vi "TouchPanel.NumericGui.vi"(4 "Password Display (F)":bool, 6 "Max Length (70)":i32=70, 8 "Integer (F)":bool, 9 "empty visible (F)":bool caption="empty visilbe (F)", 10 "Numeric In":ext, 11 "Message In":string) -> (1 "Canceled":bool, 2 "Numeric Out":ext)   [LabVIEW 2016]
uses:
  TouchPanel.DriverCommands.ctl
  Translator/Translator.Global.vi
panel:
  in  "Empty":bool
  in  "~-Inf":bool caption="-Inf"
  in  "~+Inf":bool caption="+Inf"
  out "Text 2":string
  out "_tab":enum32{"Keyboard", "Arrows"}(tab)
  in  "~.":bool
  in  "~0":bool
  in  "~9":bool
  in  "~8":bool
  in  "~7":bool
  in  "~6":bool
  in  "~5":bool
  in  "~4":bool
  in  "~3":bool
  in  "~2":bool
  in  "~1":bool
  in  "~UP":bool
  in  "~Down":bool
  in  "~-":bool caption="-"
  in  "~+":bool caption="+"
  in  "~Right":bool
  in  "~Left":bool
  in  "Clear":bool
  in  "~+/-":bool
  out "Message":string
  in  "OKButton":bool
  in  "CancelButton":bool
  in  "Text":string
  in  "Delete":bool
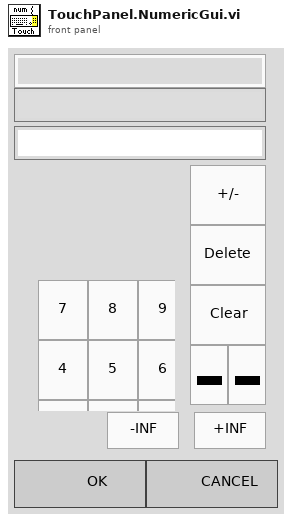
[diagram p1: front panel]
types:
  T1 = typedef "TouchPanel.DriverCommands.ctl" = enum16{"No Command", "Initialize", "Add Character", "Replace Character", "Delete Character", "Move Left", "Move Right", "Update Edit Position"}
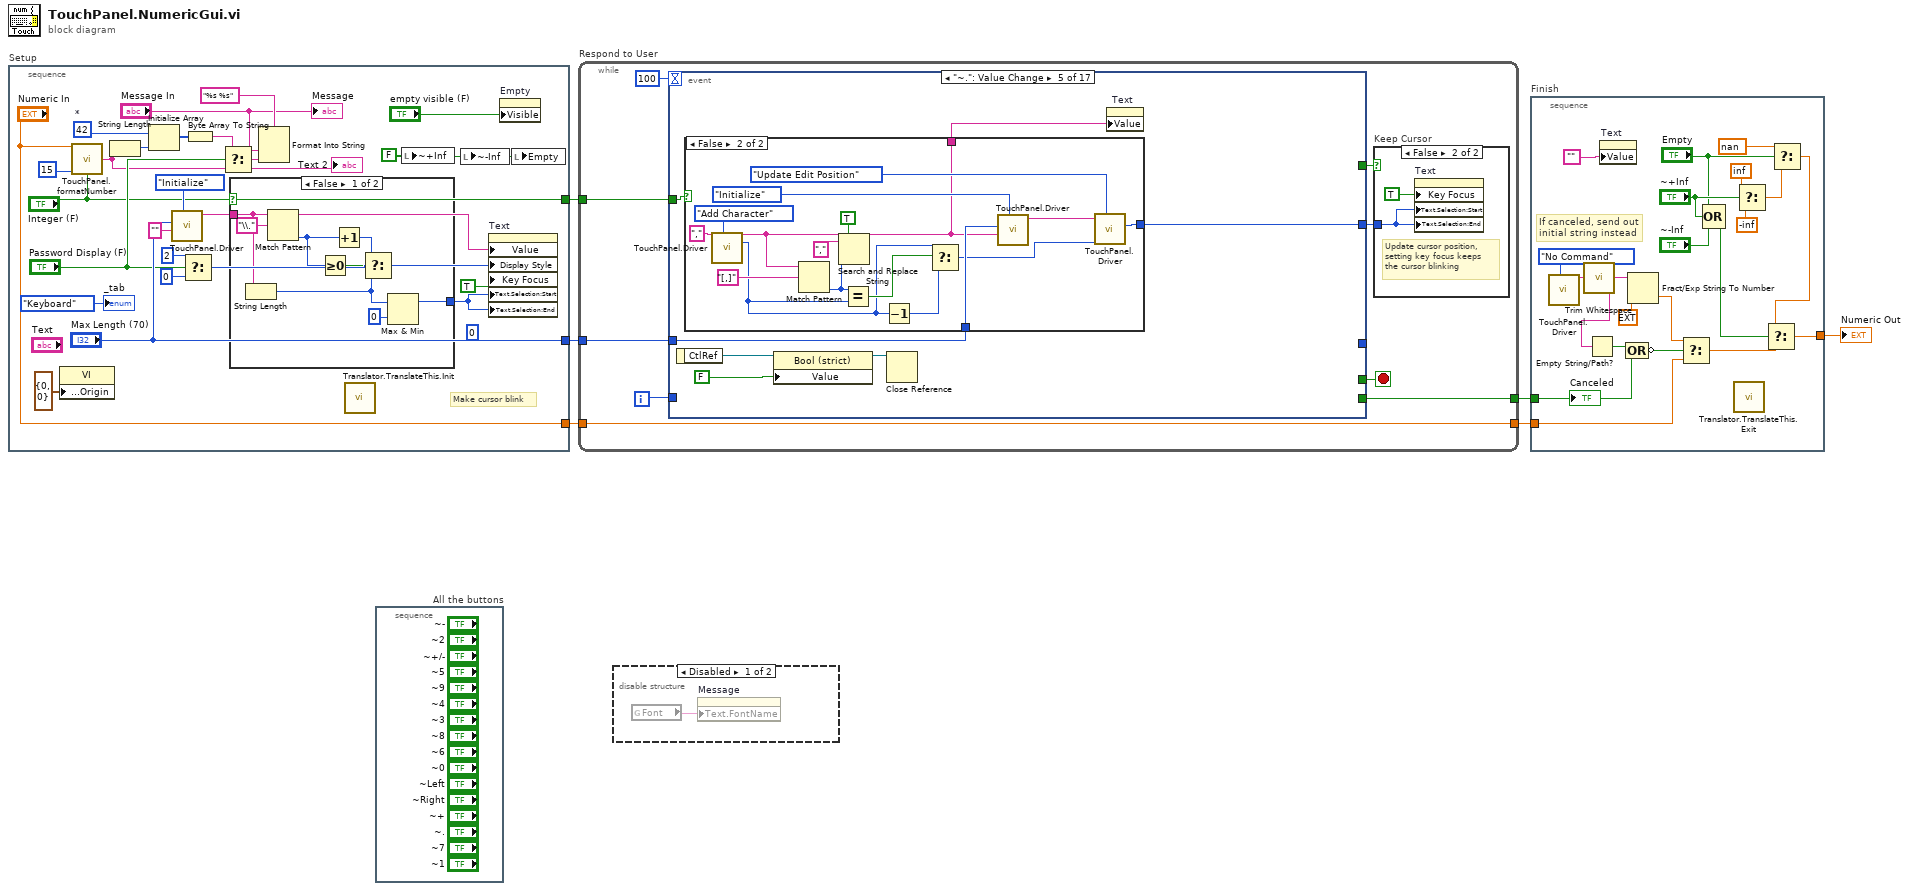
[diagram p0: block diagram]
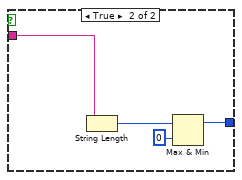
[diagram p3: hidden frame]
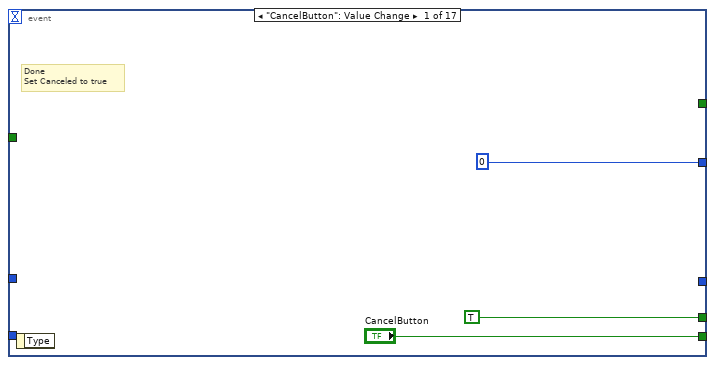
[diagram p5: hidden frame]
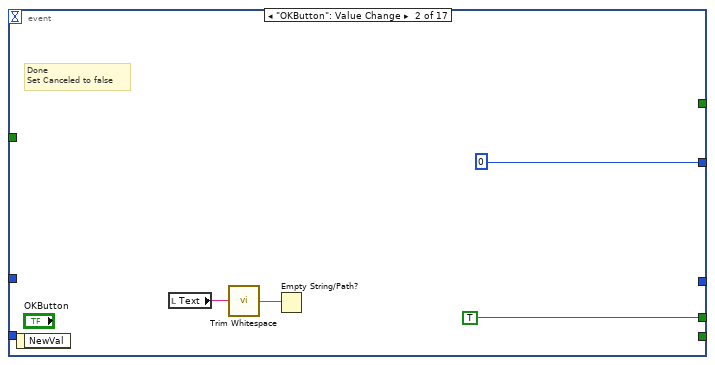
[diagram p6: hidden frame]
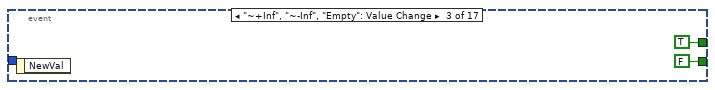
[diagram p7: hidden frame]
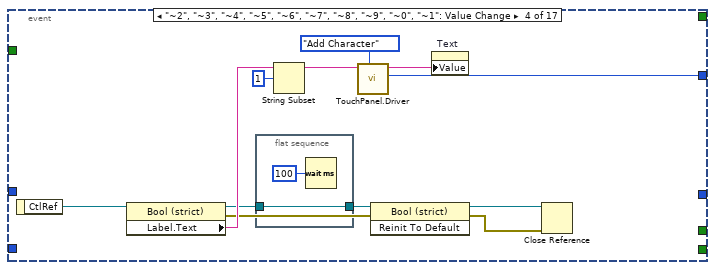
[diagram p8: hidden frame]
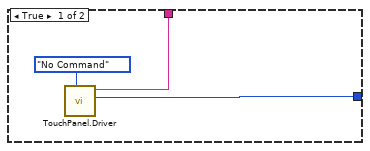
[diagram p9: hidden frame]
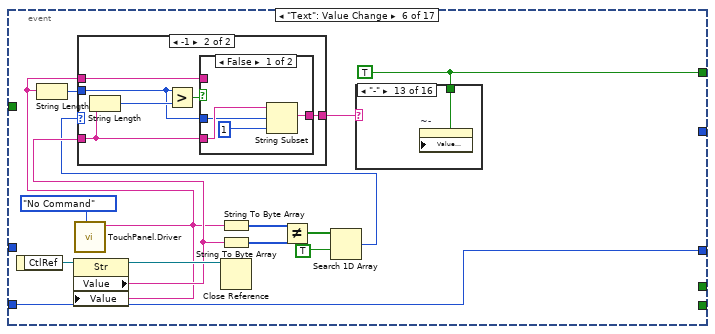
[diagram p10: hidden frame]
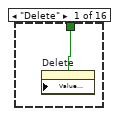
[diagram p11: hidden frame]
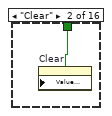
[diagram p12: hidden frame]
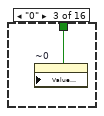
[diagram p13: hidden frame]
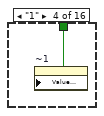
[diagram p14: hidden frame]
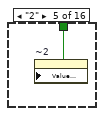
[diagram p15: hidden frame]
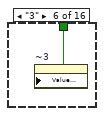
[diagram p16: hidden frame]
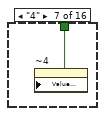
[diagram p17: hidden frame]
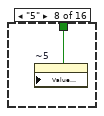
[diagram p18: hidden frame]
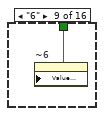
[diagram p19: hidden frame]
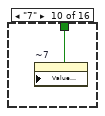
[diagram p20: hidden frame]
diagram:
  n1 = stacked-sequence "Setup" {
    tunnel: ["Numeric In"] -> w6
    tunnel: ["Max Length (70)"] -> w3
    tunnel: ["Integer (F)"] -> w2
    frame #0 {
      w8 = FALSE ("+Inf")
      (unwired) u32 0 ("Text.Selection:End")
      w19 = u8 42  # *
      # "Make cursor blink"
      n2 = property class="VI"("Front Panel Window:Origin"=cluster{"Horizontal":i16, "Vertical":i16} {"Horizontal"=0, "Vertical"=0}) -> ()  [unwired: 2 in, 2 out]
      n3 = call "TouchPanel.formatNumber.vi"("number in"="Numeric In", "significant digits (6)"=i16 15, "Integer (F)"="Integer (F)") -> ("string out"=w9:string)  [unwired: 1 in, 11 out]
      "Text 2" <- w9
      n4 = String Length(string=w9) -> (length=w20:i32)
      n5 = Initialize Array(w19, w20) -> (w18:u8[])
      n6 = call "TouchPanel.Driver.vi"("Driver Commands"=TouchPanel.DriverCommands."Initialize", "Initial String"="", "Max Length (70)"="Max Length (70)") -> ("String Out"=w12:string)  [unwired: 2 in, 6 out]
      n7 = Select(t=u32 2 ("Display Style"), s="Password Display (F)", f=u32 0 ("Display Style")) -> (s? t:f=w28:u32)
      n8 = Byte Array To String(unsigned byte array=w18) -> (string=w17:string)
      n9 = Select(t=w17, s="Password Display (F)", f=w9) -> (s? t:f=w22:string)
      n10 = case shown="False" "Integer (F)" {
        tunnel: w12 -> [w37 w43]
        tunnel: [w35 w42] -> w11
        frame False {
          n11 = String Length(string=w37) -> (length=w32:i32)
          n12 = Match Pattern(string=w37, regular expression="\\.") -> (offset past match=w34:i32)  [unwired: 4 out]
          n13 = Greater Or Equal To 0?(x=w34) -> (x >= 0?=w38:bool)
          n14 = Increment(x=w34) -> (x+1=w33:i32)
          n15 = Select(t=w33, s=w38, f=w32) -> ()  [unwired: 1 out]
          n16 = Max & Min(x=w32, y=0 ("Text.Selection:End")) -> (max(x,y)=w35:i32)  [unwired: 1 out]
        }
        frame True {
          n17 = String Length(string=w43) -> (length=w40:i32)
          n18 = Max & Min(x=w40, y=0 ("Text.Selection:End")) -> (max(x,y)=w42:i32)  [unwired: 1 out]
        }
      }
      n19 = Format Into String(format string="%s %s", "Message In", w22) -> ()  [unwired: 2 in, 2 out]
      n20 = call "Translator.TranslateThis.Init.vi"() -> ()  [unwired: 11 in, 1 out]
      n21 = local write "~+Inf"(w8) -> ()
      n22 = local write "~-Inf"(w8) -> ()
      n23 = property on="Text" class="Str"("Value"=w12, "Display Style"=w28, "Key Focus"=TRUE, "Text.Selection:Start"=w11, "Text.Selection:End"=w11) -> ()  [unwired: 2 in, 2 out]
      n24 = property on="Empty" class="Bool (strict)"("Visible"="empty visible (F)") -> ()  [unwired: 2 in, 2 out]
      n25 = local write "Empty"(w8) -> ()
      "Message" <- "Message In"
      "_tab" <- enum32{"Keyboard", "Arrows"}."Keyboard" ("_tab")
    }
  }
  n26 = stacked-sequence "All the buttons" {
    frame #0 {
    }
  }
  n27 = while "Respond to User" {
    tunnel: w6 -> [w49]
    tunnel: [w50] -> w5
    tunnel: [w49] -> w4
    tunnel: w3 -> [w48]
    tunnel: w2 -> [w44]
    i -> [w45]
    stop <- w52 stop-if-true
    n28 = event shown="[4] \"~.\": Value Change" {
      selector: _ -> [_ _ _ _ _ _ _ _ _ _ _ _ _ _ _ _ _]
      dyn-events: _ -> [_ _ _ _ _ _ _ _ _ _ _ _ _ _ _ _ _]
      timeout: 100 -> [_ _ _ _ _ _ _ _ _ _ _ _ _ _ _ _ _]
      tunnel: [TRUE TRUE TRUE _ _ _ _ _ _ _ _ _ _ _ _ _ _] -> w52
      tunnel: [0 ("Edit Position") 0 ("Edit Position") _ w72 w84 _ _ w173 w198 w220 u32 0 ("Text.Selection Start") w241 w263 w273 w337 w401 w403] -> w51
      tunnel: ["CancelButton" _ FALSE ("Cancel") _ _ _ _ _ _ _ _ _ _ _ _ _ _] -> w50
      tunnel: w48 -> [_ _ _ _ w83 _ _ w176 w201 w223 w238 _ _ w294 w360 _ _]
      tunnel: [_ _ _ _ _ w108 TRUE _ _ _ _ _ _ _ _ _ _] -> w47
      tunnel: w45 -> [_ _ _ _ _ w107 _ _ _ _ _ _ _ _ _ _ _]
      tunnel: [_ _ _ _ _ w107 _ _ _ _ _ _ _ _ _ _ _] -> _
      tunnel: w44 -> [_ _ _ _ w78 _ _ _ _ _ _ _ _ w286 w351 _ _]
      event "CancelButton": Value Change {
        # "Done\nSet Canceled to true"
        n29 = event-data() -> ()  [unwired: 2 out]
      }
      event "OKButton": Value Change {
        # "Done\nSet Canceled to false"
        n30 = event-data() -> ()  [unwired: 2 out]
        n31 = local read "Text"() -> (w58:string)
        n32 = call <vilib>:"Trim Whitespace.vi"("string"=w58) -> ("trimmed string"=w59:string)  [unwired: 1 in]
        n33 = Empty String/Path?(string/path=w59) -> ()  [unwired: 1 out]
      }
      event "~+Inf", "~-Inf", "Empty": Value Change {
        n34 = event-data() -> ()  [unwired: 2 out]
      }
      event "~2", "~3", "~4", "~5", "~6", "~7", "~8", "~9", "~0", "~1": Value Change {
        n35 = event-data() -> ("CtlRef"=w75:refnum<vi>)  [unwired: 1 out]
        n36 = property class="Bool (strict)"(reference=w75) -> (reference out=w67:refnum<vi>, error out=w65:errorcluster, "Label.Text"=w73:string)  [unwired: 1 in]
        n37 = flat-sequence {
          tunnel: [w77] -> w66
          tunnel: w67 -> [w77]
          frame #0 {
            n38 = Wait (ms)(milliseconds to wait=u32 100) -> ()  [unwired: 1 out]
          }
        }
        n39 = String Subset(string=w73, offset (0)=1) -> (substring=w70:string)  [unwired: 1 in]
        n40 = call "TouchPanel.Driver.vi"("Driver Commands"=TouchPanel.DriverCommands."Add Character", "Character"=w70) -> ("Edit Position"=w72:i32, "String Out"=w71:string)  [unwired: 3 in, 5 out]
        n41 = invoke class="Bool (strict)" method="Reinit To Default"(reference=w66, error in=w65) -> (reference out=w68:refnum<vi>, error out=w64:errorcluster)  [unwired: 1 in, 1 out]
        n42 = property on="Text" class="Str"("Value"=w71) -> ()  [unwired: 2 in, 2 out]
        n43 = Close Reference(reference=w68, error in (no error)=w64) -> ()  [unwired: 1 out]
      }
      event "~.": Value Change {
        n44 = event-data() -> ("CtlRef"=w80:refnum<vi>)  [unwired: 1 out]
        n45 = case shown="False" w78 {
          tunnel: [w86 w101] -> w84
          tunnel: w83 -> [_ w100]
          tunnel: [w85 w88] -> w79
          frame True {
            n46 = call "TouchPanel.Driver.vi"("Driver Commands"=TouchPanel.DriverCommands."No Command") -> ("Edit Position"=w86:i32, "String Out"=w85:string)  [unwired: 4 in, 5 out]
          }
          frame False {
            n47 = call "TouchPanel.Driver.vi"("Driver Commands"=TouchPanel.DriverCommands."Add Character", "Character"=",") -> ("Edit Position"=w90:i32, "String Out"=w96:string)  [unwired: 3 in, 5 out]
            n48 = Match Pattern(string=w96, regular expression="[,]") -> (offset past match=w92:i32)  [unwired: 4 out]
            n49 = Search and Replace String(replace all?=TRUE ("replace all? (F)"), input string=w96, search string="," ("Character"), offset=w92) -> (result string=w88:string)  [unwired: 1 in, 6 out]
            n50 = Equal?(x=w92, y=w90) -> (x = y?=w91:bool)
            n51 = Decrement(x=w90) -> (x-1=w89:i32)
            n52 = Select(t=w90, s=w91, f=w89) -> (s? t:f=w93:i32)
            n53 = call "TouchPanel.Driver.vi"("Driver Commands"=TouchPanel.DriverCommands."Initialize", "Initial String"=w88, "Max Length (70)"=w100) -> ("String Out"=w103:string)  [unwired: 2 in, 6 out]
            n54 = call "TouchPanel.Driver.vi"("Driver Commands"=TouchPanel.DriverCommands."Update Edit Position", "New Edit Position"=w93, "Character"=w103) -> ("Edit Position"=w101:i32)  [unwired: 2 in, 6 out]
          }
        }
        n55 = property class="Bool (strict)"(reference=w80, "Value"=FALSE) -> (reference out=w82:refnum<vi>)  [unwired: 1 in, 1 out]
        n56 = Close Reference(reference=w82) -> ()  [unwired: 1 in, 1 out]
        n57 = property on="Text" class="Str"("Value"=w79) -> ()  [unwired: 2 in, 2 out]
      }
      event "Text": Value Change {
        w108 = TRUE
        n58 = event-data() -> ("CtlRef"=w118:refnum<vi>)  [unwired: 1 out]
        n59 = call "TouchPanel.Driver.vi"("Driver Commands"=TouchPanel.DriverCommands."No Command") -> ("String Out"=w106:string)  [unwired: 4 in, 6 out]
        n60 = String Length(string=w106) -> (length=w115:i32)
        n61 = property class="Str"(reference=w118, "Value"=w106) -> (reference out=w117:refnum<vi>, "Value"=w111:string)  [unwired: 1 in, 1 out]
        n62 = String To Byte Array(string=w106) -> (unsigned byte array=w112:u8[])
        n63 = String To Byte Array(string=w111) -> (unsigned byte array=w113:u8[])
        n64 = Close Reference(reference=w117) -> ()  [unwired: 1 in, 1 out]
        n65 = Not Equal?(x=w112, y=w113) -> (x != y?=w110:bool[])
        n66 = Search 1D Array(1D array=w110, element=TRUE) -> (index of element=w105:i32)  [unwired: 1 out]
        n67 = case shown="-1" w105 {
          selector: w105 -> [w135 _]
          tunnel: w106 -> [w137 w150]
          tunnel: w111 -> [w136 w149]
          tunnel: w115 -> [w139 w146]
          tunnel: [w134 w148] -> w109
          frame Default {
            n68 = String Length(string=w136) -> (length=w140:i32)
            n69 = Greater?(x=w139, y=w140) -> (0:w138:bool)
            n70 = case shown="False" w138 {
              tunnel: w137 -> [_ _]
              tunnel: w136 -> [w144 _]
              tunnel: w135 -> [w143 _]
              tunnel: [w141 "Delete" ("Value")] -> w134
              frame False {
                n71 = String Subset(string=w144, offset (0)=w143, length (rest)=1 ("length (rest)")) -> (substring=w141:string)
              }
              frame True {
              }
            }
          }
          frame -1 {
            n72 = String Length(string=w149) -> (length=w147:i32)
            n73 = Greater?(x=w146, y=w147) -> (0:w151:bool)
            n74 = case shown="False" w151 {
              tunnel: w150 -> [_ _]
              tunnel: w149 -> [w155 _]
              tunnel: w146 -> [w154 _]
              tunnel: [w152 "Delete" ("Value")] -> w148
              frame False {
                n75 = String Subset(string=w155, offset (0)=w154, length (rest)=1 ("length (rest)")) -> (substring=w152:string)
              }
              frame True {
              }
            }
          }
        }
        n76 = case shown="\"-\"" w109 {
          tunnel: w108 -> [w119 w120 w121 w122 w123 w124 w125 w126 w127 w128 w129 w130 w131 w132 w133 _]
          frame "Delete" {
            n77 = property on="Delete" class="Bool (strict)"("Value (Signaling)"=w119) -> ()  [unwired: 2 in, 2 out]
          }
          frame "Clear" {
            n78 = property on="Clear" class="Bool (strict)"("Value (Signaling)"=w120) -> ()  [unwired: 2 in, 2 out]
          }
          frame "0" {
            n79 = property on="~0" class="Bool (strict)"("Value (Signaling)"=w121) -> ()  [unwired: 2 in, 2 out]
          }
          frame "1" {
            n80 = property on="~1" class="Bool (strict)"("Value (Signaling)"=w122) -> ()  [unwired: 2 in, 2 out]
          }
          frame "2" {
            n81 = property on="~2" class="Bool (strict)"("Value (Signaling)"=w123) -> ()  [unwired: 2 in, 2 out]
          }
          frame "3" {
            n82 = property on="~3" class="Bool (strict)"("Value (Signaling)"=w124) -> ()  [unwired: 2 in, 2 out]
          }
          frame "4" {
            n83 = property on="~4" class="Bool (strict)"("Value (Signaling)"=w125) -> ()  [unwired: 2 in, 2 out]
          }
          frame "5" {
            n84 = property on="~5" class="Bool (strict)"("Value (Signaling)"=w126) -> ()  [unwired: 2 in, 2 out]
          }
          frame "6" {
            n85 = property on="~6" class="Bool (strict)"("Value (Signaling)"=w127) -> ()  [unwired: 2 in, 2 out]
          }
          frame "7" {
            n86 = property on="~7" class="Bool (strict)"("Value (Signaling)"=w128) -> ()  [unwired: 2 in, 2 out]
          }
          frame "8" {
            n87 = property on="~8" class="Bool (strict)"("Value (Signaling)"=w129) -> ()  [unwired: 2 in, 2 out]
          }
          frame "9" {
            n88 = property on="~9" class="Bool (strict)"("Value (Signaling)"=w130) -> ()  [unwired: 2 in, 2 out]
          }
          frame "-" {
            n89 = property on="~-" class="Bool (strict)"("Value (Signaling)"=w131) -> ()  [unwired: 2 in, 2 out]
          }
          frame "+" {
            n90 = property on="~+" class="Bool (strict)"("Value (Signaling)"=w132) -> ()  [unwired: 2 in, 2 out]
          }
          frame "." {
            n91 = property on="~." class="Bool (strict)"("Value (Signaling)"=w133) -> ()  [unwired: 2 in, 2 out]
          }
          frame Default {
          }
        }
      }
      event Timeout {
        n92 = event-data() -> ()  [unwired: 2 out]
        n93 = property on="Text" class="Str"() -> ("Text.Selection:Start"=w158:u32)  [unwired: 2 in, 2 out]
        n94 = call "TouchPanel.Driver.vi"("Driver Commands"=TouchPanel.DriverCommands."No Command") -> ("Edit Position"=w160:i32)  [unwired: 4 in, 6 out]
        n95 = Not Equal?(x=w160, y=w158) -> (x != y?=w159:bool)
        n96 = case shown="True" w159 {
          tunnel: w158 -> [_ w162]
          frame False {
          }
          frame True {
            n97 = call "TouchPanel.Driver.vi"("Driver Commands"=TouchPanel.DriverCommands."Update Edit Position", "New Edit Position"=w162) -> ()  [unwired: 3 in, 7 out]
          }
        }
      }
      event "~+/-": Value Change {
        w170 = "-" ("regular expression")
        n98 = event-data() -> ("CtlRef"=w166:refnum<vi>)  [unwired: 1 out]
        n99 = property on="Text" class="Str"() -> ("Value"=w171:string, "Text.Selection:Start"=w169:u32)  [unwired: 2 in, 2 out]
        n100 = property class="Bool (strict)"(reference=w166, "Value"=FALSE) -> (reference out=w168:refnum<vi>)  [unwired: 1 in, 1 out]
        n101 = Match Pattern(string=w171, regular expression=w170) -> (offset past match=w172:i32)  [unwired: 4 out]
        n102 = Close Reference(reference=w168) -> ()  [unwired: 1 in, 1 out]
        n103 = case shown="Default" w172 {
          selector: w172 -> [w180 _]
          tunnel: w171 -> [w182 w187]
          tunnel: w170 -> [_ w186]
          tunnel: w169 -> [w181 w185]
          tunnel: [w179 w184] -> w164
          tunnel: [w178 w183] -> w165
          frame Default {
            n104 = String Subset(string=w182, offset (0)=w180) -> (substring=w178:string)  [unwired: 1 out]
            n105 = Subtract(x=w181, y=w180) -> (x-y=w179:u32)
          }
          frame -1 {
            n106 = Increment(x=w185) -> (x+1=w184:u32)
            n107 = Concatenate Strings(w186, w187) -> (w183:string)
          }
        }
        n108 = call "TouchPanel.Driver.vi"("Driver Commands"=TouchPanel.DriverCommands."Initialize", "Initial String"=w165, "Max Length (70)"=w176) -> ("String Out"=w175:string)  [unwired: 2 in, 6 out]
        n109 = property on="Text" class="Str"("Value"=w165) -> ()  [unwired: 2 in, 2 out]
        n110 = call "TouchPanel.Driver.vi"("Driver Commands"=TouchPanel.DriverCommands."Update Edit Position", "New Edit Position"=w164, "Character"=w175) -> ("Edit Position"=w173:i32)  [unwired: 2 in, 6 out]
      }
      event "~+": Value Change {
        w196 = "-" ("regular expression")
        n111 = event-data() -> ("CtlRef"=w193:refnum<vi>)  [unwired: 1 out]
        n112 = call "TouchPanel.Driver.vi"("Driver Commands"=TouchPanel.DriverCommands."No Command") -> ("Edit Position"=w190:i32, "String Out"=w191:string)  [unwired: 4 in, 5 out]
        n113 = property class="Bool (strict)"(reference=w193, "Value"=FALSE) -> (reference out=w195:refnum<vi>)  [unwired: 1 in, 1 out]
        n114 = Match Pattern(string=w191, regular expression=w196) -> (offset past match=w197:i32)  [unwired: 4 out]
        n115 = Close Reference(reference=w195) -> ()  [unwired: 1 in, 1 out]
        n116 = case shown="Default" w197 {
          selector: w197 -> [w205 _]
          tunnel: w191 -> [w207 w209]
          tunnel: w196 -> [_ _]
          tunnel: w190 -> [w206 w208]
          tunnel: [w204 w208] -> w188
          tunnel: [w203 w209] -> w189
          frame Default {
            n117 = Subtract(x=w206, y=w205) -> (x-y=w204:i32)
            n118 = String Subset(string=w207, offset (0)=w205) -> (substring=w203:string)  [unwired: 1 out]
          }
          frame -1 {
          }
        }
        n119 = call "TouchPanel.Driver.vi"("Driver Commands"=TouchPanel.DriverCommands."Initialize", "Initial String"=w189, "Max Length (70)"=w201) -> ("String Out"=w200:string)  [unwired: 2 in, 6 out]
        n120 = property on="Text" class="Str"("Value"=w189) -> ()  [unwired: 2 in, 2 out]
        n121 = call "TouchPanel.Driver.vi"("Driver Commands"=TouchPanel.DriverCommands."Update Edit Position", "New Edit Position"=w188, "Character"=w200) -> ("Edit Position"=w198:i32)  [unwired: 2 in, 6 out]
      }
      event "~-": Value Change {
        w218 = "-" ("regular expression")
        n122 = event-data() -> ("CtlRef"=w215:refnum<vi>)  [unwired: 1 out]
        n123 = call "TouchPanel.Driver.vi"("Driver Commands"=TouchPanel.DriverCommands."No Command") -> ("Edit Position"=w212:i32, "String Out"=w213:string)  [unwired: 4 in, 5 out]
        n124 = property class="Bool (strict)"(reference=w215, "Value"=FALSE) -> (reference out=w217:refnum<vi>)  [unwired: 1 in, 1 out]
        n125 = Match Pattern(string=w213, regular expression=w218) -> (offset past match=w219:i32)  [unwired: 4 out]
        n126 = Close Reference(reference=w217) -> ()  [unwired: 1 in, 1 out]
        n127 = case shown="-1" w219 {
          tunnel: w213 -> [w226 w231]
          tunnel: w218 -> [_ w230]
          tunnel: w212 -> [w225 w229]
          tunnel: [w226 w228] -> w211
          tunnel: [w225 w227] -> w210
          frame Default {
          }
          frame -1 {
            n128 = Increment(x=w229) -> (x+1=w227:i32)
            n129 = Concatenate Strings(w230, w231) -> (w228:string)
          }
        }
        n130 = call "TouchPanel.Driver.vi"("Driver Commands"=TouchPanel.DriverCommands."Initialize", "Initial String"=w211, "Max Length (70)"=w223) -> ("String Out"=w222:string)  [unwired: 2 in, 6 out]
        n131 = property on="Text" class="Str"("Value"=w211) -> ()  [unwired: 2 in, 2 out]
        n132 = call "TouchPanel.Driver.vi"("Driver Commands"=TouchPanel.DriverCommands."Update Edit Position", "New Edit Position"=w210, "Character"=w222) -> ("Edit Position"=w220:i32)  [unwired: 2 in, 6 out]
      }
      event "Clear": Value Change {
        n133 = event-data() -> ("CtlRef"=w234:refnum<vi>)  [unwired: 1 out]
        n134 = property class="Bool (strict)"(reference=w234, "Value"=FALSE) -> (reference out=w236:refnum<vi>)  [unwired: 1 in, 1 out]
        n135 = call "TouchPanel.Driver.vi"("Driver Commands"=TouchPanel.DriverCommands."Initialize", "Initial String"="", "Max Length (70)"=w238) -> ("String Out"=w237:string)  [unwired: 2 in, 6 out]
        n136 = Close Reference(reference=w236) -> ()  [unwired: 1 in, 1 out]
        n137 = property on="Text" class="Str"("Value"=w237) -> ()  [unwired: 2 in, 2 out]
      }
      event "~Left": Value Change {
        w243 = 1 ("length (rest)")
        n138 = event-data() -> ("CtlRef"=w250:refnum<vi>)  [unwired: 1 out]
        n139 = property on="Text" class="Str"() -> ("Value"=w249:string, "Text.Selection Start"=w240:u32)  [unwired: 2 in, 2 out]
        n140 = property class="Bool (strict)"(reference=w250, "Value"=FALSE) -> (reference out=w252:refnum<vi>)  [unwired: 1 in, 1 out]
        n141 = String Subset(string=w249, offset (0)=0, length (rest)=w243) -> (substring=w247:string)
        n142 = Equal?(x=w243, y=w240) -> (x = y?=w245:bool)
        n143 = Equal?(x="-", y=w247) -> (x = y?=w244:bool)
        n144 = Compound Arithmetic op=AND(w244, w245) -> (w242:bool)
        n145 = Close Reference(reference=w252) -> ()  [unwired: 1 in, 1 out]
        n146 = case shown="False" w242 {
          tunnel: [w253 w255] -> w241
          tunnel: w240 -> [_ w255]
          frame False {
            n147 = call "TouchPanel.Driver.vi"("Driver Commands"=TouchPanel.DriverCommands."Move Left") -> ("Edit Position"=w253:i32)  [unwired: 4 in, 6 out]
          }
          frame True {
          }
        }
      }
      event "~Right": Value Change {
        n148 = event-data() -> ("CtlRef"=w260:refnum<vi>)  [unwired: 1 out]
        n149 = property on="Text" class="Str"() -> ("Value"=w259:string, "Text.Selection Start"=w257:u32)  [unwired: 2 in, 2 out]
        n150 = property class="Bool (strict)"(reference=w260, "Value"=FALSE) -> (reference out=w262:refnum<vi>)  [unwired: 1 in, 1 out]
        n151 = String Length(string=w259) -> (length=w256:i32)
        n152 = Equal?(x=w256, y=w257) -> (x = y?=w258:bool)
        n153 = case shown="False" w258 {
          tunnel: [w264 w266] -> w263
          tunnel: w257 -> [_ w266]
          frame False {
            n154 = call "TouchPanel.Driver.vi"("Driver Commands"=TouchPanel.DriverCommands."Move Right") -> ("Edit Position"=w264:i32)  [unwired: 4 in, 6 out]
          }
          frame True {
          }
        }
        n155 = Close Reference(reference=w262) -> ()  [unwired: 1 in, 1 out]
      }
      event "~UP": Value Change {
        n156 = event-data() -> ()  [unwired: 2 out]
        n157 = property on="Text" class="Str"() -> ("Value"=w290:string, "Text.Selection Start"=w268:u32)  [unwired: 2 in, 2 out]
        n158 = To Long Integer(number=w268) -> (32bit integer=w287:i32)
        n159 = String Length(string=w290) -> (length=w291:i32)
        n160 = Match Pattern(string=w290, regular expression="\\.") -> (offset past match=w292:i32)  [unwired: 4 out]
        n161 = case shown="-1" w292 {
          selector: w292 -> [_ _ w316]
          tunnel: w287 -> [w297 w311 w317]
          tunnel: [w299 w310 w321] -> w289
          tunnel: w291 -> [w298 w312 _]
          tunnel: w286 -> [_ w309 w315]
          frame 0 {
            n162 = Subtract(x=w298, y=w297) -> (x-y=w302:i32)
            n163 = Subtract(x=w302, y=1) -> (x-y=w300:i32)
            n164 = Power Of 10(x=w300) -> (10^x=w299:dbl)
          }
          frame -1 {
            n165 = Subtract(x=w312, y=w311) -> (x-y=w307:i32)
            n166 = Subtract(x=w307, y=1) -> (x-y=w313:i32)
            n167 = Equal To 0?(x=w307) -> (x = 0?=w306:bool)
            n168 = Power Of 10(x=w313) -> (10^x=w308:dbl)
            n169 = To Long Integer(number=w308) -> (32bit integer=w304:i32)
            n170 = Select(t=1, s=w306, f=w304) -> (s? t:f=w305:i32)
            n171 = Select(t=w305, s=w309, f=w308) -> (s? t:f=w310:dbl)
          }
          frame Default {
            n172 = Decrement(x=w316) -> (x-1=w318:i32)
            n173 = Greater Or Equal?(x=w317, y=w316) -> (x >= y?=w319:bool)
            n174 = Equal?(x=w318, y=w317) -> (x = y?=w320:bool)
            n175 = case shown="False" w320 {
              tunnel: w317 -> [w330 _]
              tunnel: [w327 0.1] -> w321
              tunnel: w316 -> [w326 _]
              tunnel: w319 -> [w325 _]
              tunnel: w315 -> [_ _]
              frame False {
                n176 = Subtract(x=w326, y=w330) -> (x-y=w328:i32)
                n177 = Select(t=1 ("y"), s=w325, f=2 ("y")) -> (s? t:f=w322:i32)
                n178 = Subtract(x=w328, y=w322) -> (x-y=w329:i32)
                n179 = Power Of 10(x=w329) -> (10^x=w327:dbl)
              }
              frame True {
              }
            }
          }
        }
        n180 = Fract/Exp String To Number(string=w290) -> (number=w285:dbl)  [unwired: 1 in, 3 out]
        n181 = Add(x=w285, y=w289) -> (x+y=w284:dbl)
        n182 = call "TouchPanel.formatNumber.vi"("number in"=w284, "significant digits (6)"=i16 15, "Integer (F)"=w286) -> ("string out"=w278:string)  [unwired: 1 in, 11 out]
        n183 = call "TouchPanel.Driver.vi"("Driver Commands"=TouchPanel.DriverCommands."Initialize", "Initial String"=w278, "Max Length (70)"=w294) -> ("String Out"=w295:string)  [unwired: 2 in, 6 out]
        n184 = property on="Text" class="Str"("Value"=w295) -> ()  [unwired: 2 in, 2 out]
        n185 = String Length(string=w278) -> (length=w267:i32)
        n186 = String Subset(string=w278, offset (0)=0, length (rest)=1 ("length (rest)")) -> (substring=w280:string)
        n187 = Equal?(x=w268, y=u32 1) -> (x = y?=w270:bool)
        n188 = Equal?(x="-", y=w280) -> (x = y?=w277:bool)
        n189 = Equal To 0?(x=w268) -> (x = 0?=w271:bool)
        n190 = Compound Arithmetic op=OR(w271, w270) -> (w269:bool)
        n191 = Compound Arithmetic op=AND(w269, w277) -> (w276:bool)
        n192 = Select(t=u32 1 ("lower limit"), s=w276, f=u32 0 ("lower limit")) -> (s? t:f=w272:u32)
        n193 = In Range and Coerce(upper limit=w267, x=w268, lower limit=w272) -> (coerced(x)=w273:u32)  [unwired: 1 out]
      }
      event "~Down": Value Change {
        n194 = event-data() -> ()  [unwired: 2 out]
        n195 = property on="Text" class="Str"() -> ("Value"=w349:string, "Text.Selection Start"=w336:u32)  [unwired: 2 in, 2 out]
        n196 = Search and Replace String(input string=w349, search string="-") -> ()  [unwired: 1 in, 9 out]
        n197 = To Long Integer(number=w336) -> (32bit integer=w352:i32)
        n198 = String Length(string=w349) -> (length=w356:i32)
        n199 = Match Pattern(string=w349, regular expression="\\.") -> (offset past match=w358:i32)  [unwired: 4 out]
        n200 = case shown="-1" w358 {
          selector: w358 -> [_ _ w381]
          tunnel: w352 -> [w363 w372 w382]
          tunnel: [w365 w369 w386] -> w355
          tunnel: w356 -> [w364 w371 _]
          tunnel: w351 -> [_ w370 _]
          frame 0 {
            n201 = Subtract(x=w364, y=w363) -> (x-y=w368:i32)
            n202 = Subtract(x=w368, y=1) -> (x-y=w366:i32)
            n203 = Power Of 10(x=w366) -> (10^x=w365:dbl)
          }
          frame -1 {
            n204 = Subtract(x=w371, y=w372) -> (x-y=w377:i32)
            n205 = Subtract(x=w377, y=1) -> (x-y=w379:i32)
            n206 = Equal To 0?(x=w377) -> (x = 0?=w376:bool)
            n207 = Power Of 10(x=w379) -> (10^x=w378:dbl)
            n208 = To Long Integer(number=w378) -> (32bit integer=w374:i32)
            n209 = Select(t=1, s=w376, f=w374) -> (s? t:f=w375:i32)
            n210 = Select(t=w375, s=w370, f=w378) -> (s? t:f=w369:dbl)
          }
          frame Default {
            n211 = Decrement(x=w381) -> (x-1=w383:i32)
            n212 = Greater Or Equal?(x=w382, y=w381) -> (x >= y?=w384:bool)
            n213 = Equal?(x=w383, y=w382) -> (x = y?=w385:bool)
            n214 = case shown="True" w385 {
              tunnel: w382 -> [w395 _]
              tunnel: [w392 0.1] -> w386
              tunnel: w381 -> [w391 _]
              tunnel: w384 -> [w390 _]
              frame False {
                n215 = Subtract(x=w391, y=w395) -> (x-y=w393:i32)
                n216 = Select(t=1 ("y"), s=w390, f=2 ("y")) -> (s? t:f=w387:i32)
                n217 = Subtract(x=w393, y=w387) -> (x-y=w394:i32)
                n218 = Power Of 10(x=w394) -> (10^x=w392:dbl)
              }
              frame True {
              }
            }
          }
        }
        n219 = Fract/Exp String To Number(string=w349) -> (number=w354:dbl)  [unwired: 1 in, 3 out]
        n220 = Subtract(x=w354, y=w355) -> (x-y=w357:dbl)
        n221 = call "TouchPanel.formatNumber.vi"("number in"=w357, "significant digits (6)"=i16 15, "Integer (F)"=w351) -> ("string out"=w338:string)  [unwired: 1 in, 11 out]
        n222 = call "TouchPanel.Driver.vi"("Driver Commands"=TouchPanel.DriverCommands."Initialize", "Initial String"=w338, "Max Length (70)"=w360) -> ("String Out"=w361:string)  [unwired: 2 in, 6 out]
        n223 = property on="Text" class="Str"("Value"=w361) -> ()  [unwired: 2 in, 2 out]
        n224 = String Length(string=w338) -> (length=w332:i32)
        n225 = String Subset(string=w338, offset (0)=0, length (rest)=1 ("length (rest)")) -> (substring=w342:string)
        n226 = Equal?(x=w336, y=u32 1) -> (x = y?=w335:bool)
        n227 = Equal To 0?(x=w336) -> (x = 0?=w334:bool)
        n228 = Equal?(x="-", y=w342) -> (x = y?=w344:bool)
        n229 = Compound Arithmetic op=OR(w334, w335) -> (w333:bool)
        n230 = Compound Arithmetic op=AND(w333, w344) -> (w345:bool)
        n231 = Select(t=u32 1 ("lower limit"), s=w345, f=u32 0 ("lower limit")) -> (s? t:f=w348:u32)
        n232 = In Range and Coerce(upper limit=w332, x=w336, lower limit=w348) -> (coerced(x)=w337:u32)  [unwired: 1 out]
      }
      event "Delete": Value Change {
        # "Delete character to the left of the edit point"
        n233 = event-data() -> ("CtlRef"=w397:refnum<vi>)  [unwired: 1 out]
        n234 = property class="Bool (strict)"(reference=w397, "Value"=FALSE) -> (reference out=w399:refnum<vi>)  [unwired: 1 in, 1 out]
        n235 = call "TouchPanel.Driver.vi"("Driver Commands"=TouchPanel.DriverCommands."Delete Character") -> ("Edit Position"=w401:i32, "String Out"=w400:string)  [unwired: 4 in, 5 out]
        n236 = property on="Text" class="Str"("Value"=w400) -> ()  [unwired: 2 in, 2 out]
        n237 = Close Reference(reference=w399) -> ()  [unwired: 1 in, 1 out]
      }
      event "Text": Mouse Up {
        # "The user changed the edit position\nby clicking in the text box"
        n238 = event-data() -> ("CtlRef"=w406:refnum<vi>)  [unwired: 1 out]
        n239 = property class="Str"(reference=w406) -> ("Text.Selection:Start"=w405:u32)  [unwired: 1 in, 2 out]
        n240 = call "TouchPanel.Driver.vi"("Driver Commands"=TouchPanel.DriverCommands."Update Edit Position", "New Edit Position"=w405) -> ("Edit Position"=w403:i32)  [unwired: 3 in, 6 out]
      }
    }
    n241 = case "Keep Cursor" shown="False" w47 {
      tunnel: w51 -> [_ w53]
      frame True {
      }
      frame False {
        # "Update cursor position,\nsetting key focus keeps\nthe cursor blinking"
        n242 = property on="Text" class="Str"("Key Focus"=TRUE, "Text.Selection:Start"=w53, "Text.Selection:End"=w53) -> ()  [unwired: 2 in, 2 out]
      }
    }
  }
  n243 = disable-structure shown="Disabled" {
    frame Disabled {
      n244 = global read "Translator.Global.vi" "Font"() -> (w407:string)
      n245 = property on="Message" class="Str"("Text.FontName"=w407) -> ()  [unwired: 2 in, 2 out]
    }
    frame Enabled {
    }
  }
  n246 = stacked-sequence "Finish" {
    tunnel: w5 -> [w411]
    tunnel: w4 -> [w427]
    tunnel: [w418] -> w1
    frame #0 {
      # "If canceled, send out\ninitial string instead"
      n247 = call "TouchPanel.Driver.vi"("Driver Commands"=TouchPanel.DriverCommands."No Command") -> ("String Out"=w410:string)  [unwired: 4 in, 6 out]
      n248 = call <vilib>:"Trim Whitespace.vi"("string"=w410) -> ("trimmed string"=w409:string)  [unwired: 1 in]
      n249 = Empty String/Path?(string/path=w409) -> (empty?=w408:bool)
      n250 = property on="Text" class="Str"("Value"="") -> ()  [unwired: 2 in, 2 out]
      n251 = Compound Arithmetic op=OR(w408, w411) -> (invert w412:bool)
      n252 = Fract/Exp String To Number(string=w409, default (0 dbl)=ext 0.0 ("default (0 DBL)")) -> (number=w425:ext)  [unwired: 1 in, 2 out]
      n253 = Select(t=w425, s=w412, f=w427) -> (s? t:f=w422:ext)
      n254 = Compound Arithmetic op=OR("Empty", "~+Inf", "~-Inf") -> (w421:bool)
      n255 = call "Translator.TranslateThis.Exit.vi"() -> ()  [unwired: 11 in, 1 out]
      n256 = Select(t=inf, s="~+Inf", f=-inf) -> (s? t:f=w416:dbl)
      n257 = Select(t=nan, s="Empty", f=w416) -> (s? t:f=w413:dbl)
      n258 = Select(t=w413, s=w421, f=w422) -> (s? t:f=w418:ext)
      "Canceled" <- w411
    }
  }
  "Numeric Out" <- w1
